vi "zipToxml.vi"(4 "passYield":dbl, 5 "DBSet":T1, 6 "uploadPath":path, 7 "successxmlpath":path, 8 "转换失败路径":path, 9 "目标路径":path, 10 "status msg ref":refnum<vi>, 11 "path":path caption="zip path") -> ()   [LabVIEW 2011]
panel:
  out "customerPN":string
  out "usedSN":string
  out "result":string
  out "upload":bool
  out "archive name out":path
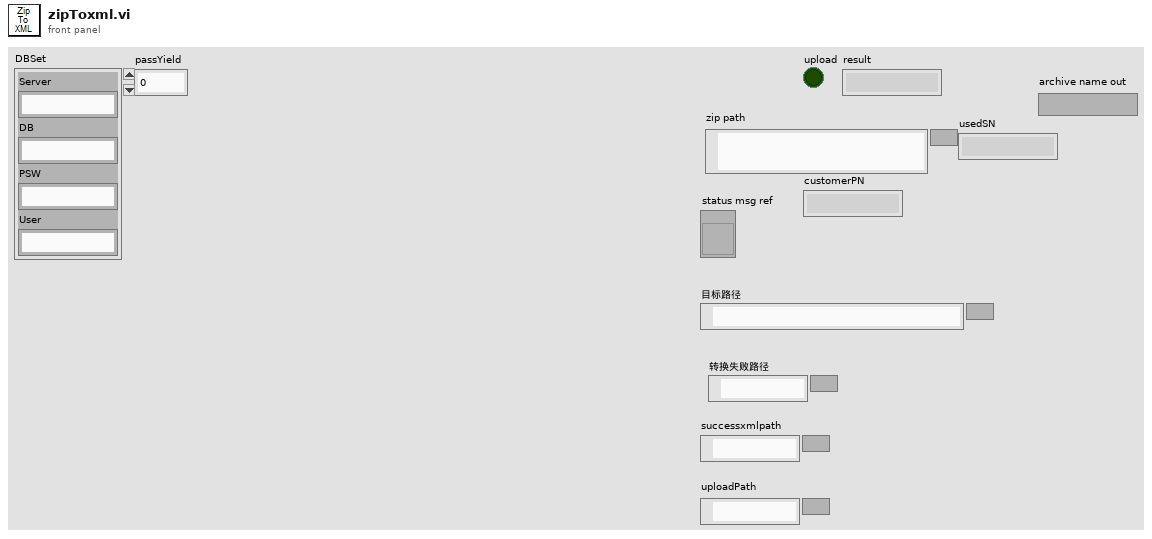
[diagram p1: front panel]
types:
  T1 = cluster{"Server":string, "DB":string, "PSW":string, "User":string}
  T2 = typedef "TDD.ctl" = cluster{"show_Cable Point":dbl[], "show_Terminal Point":dbl[], "show_impspec":string[]}
  T3 = typedef "xml_detail.ctl" = cluster{"FileVersion":string, "FileName":string, "customerPN":string, "usedSN":string, "test time":string[], "testResult":bool}
  T4 = typedef "sSpec.ctl" = cluster{"itemName":string, "upperLimit":dbl[], "lowerLimit":dbl[], "testResult":string, "result":bool}
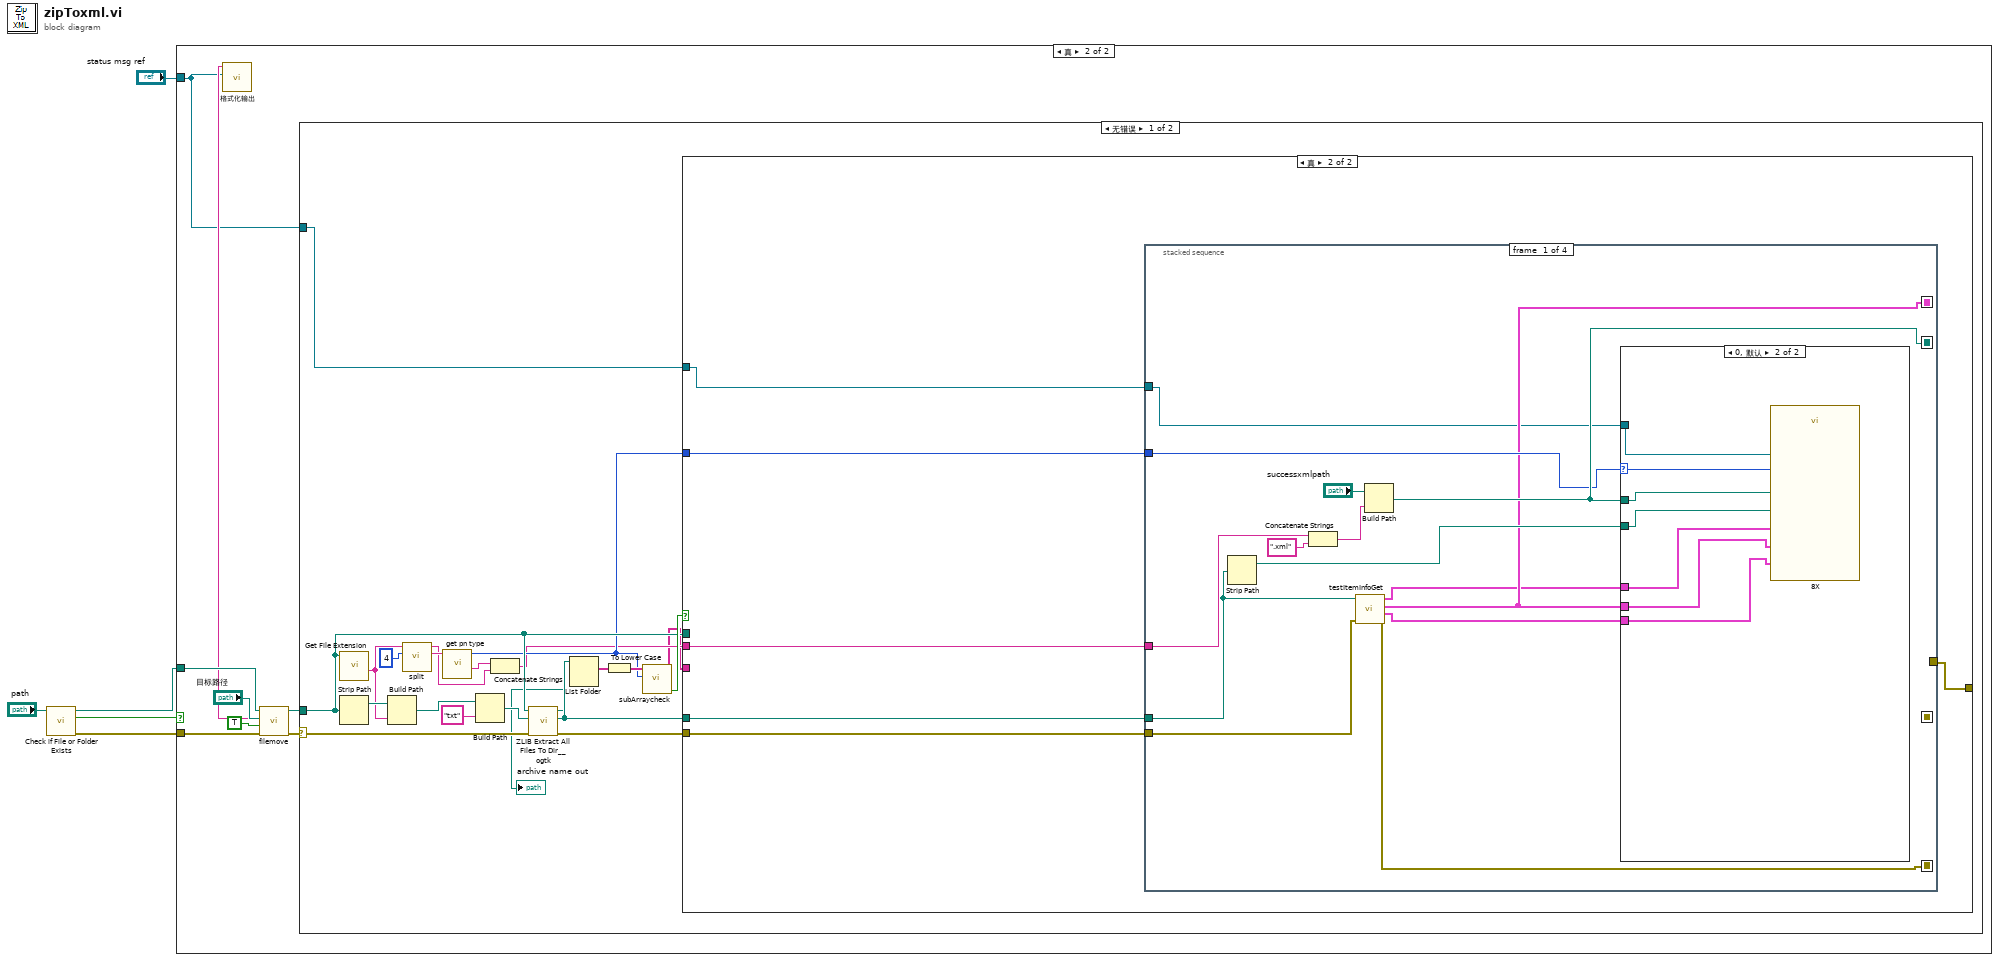
[diagram p0: block diagram]
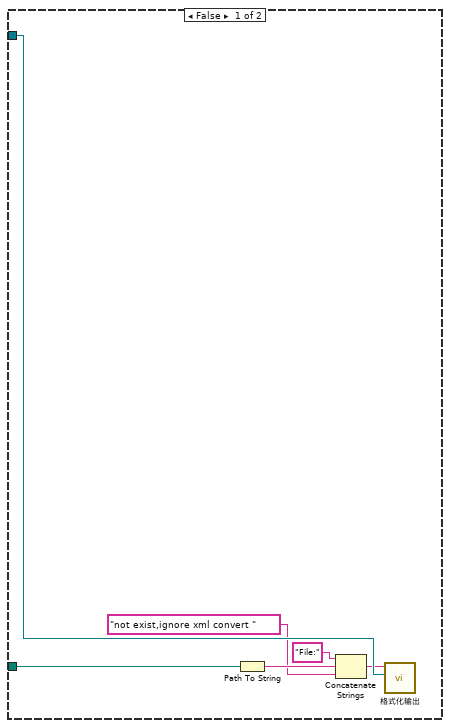
[diagram p2: hidden frame]
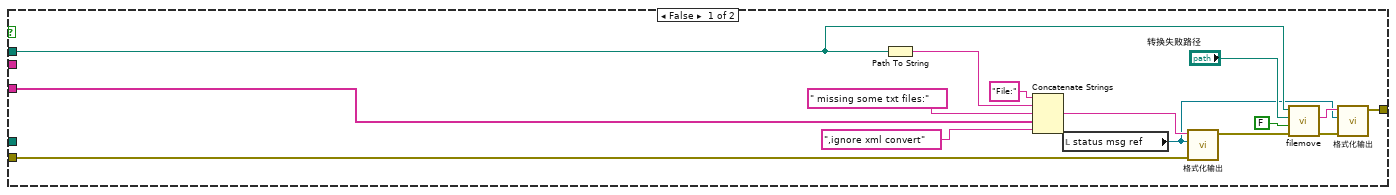
[diagram p3: hidden frame]
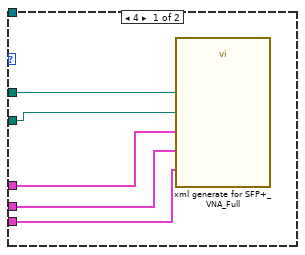
[diagram p4: hidden frame]
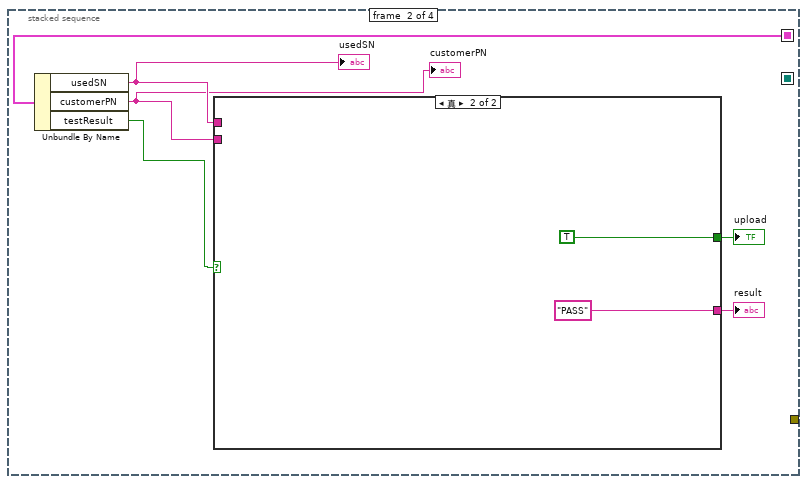
[diagram p5: hidden frame]
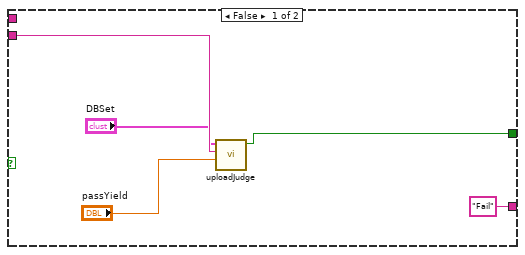
[diagram p6: hidden frame]
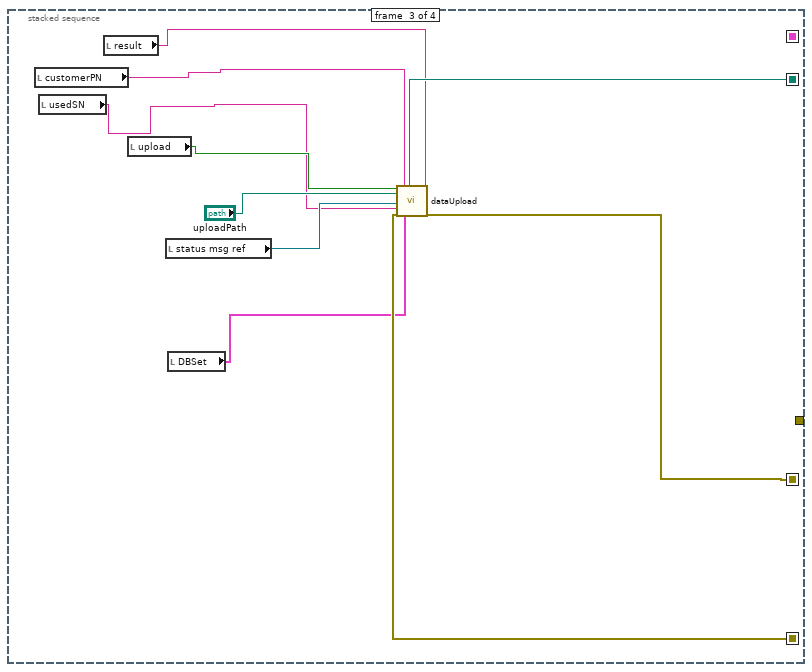
[diagram p7: hidden frame]
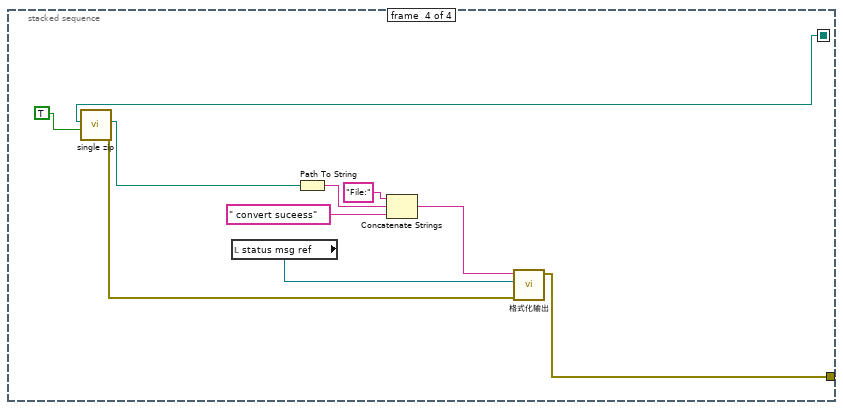
[diagram p8: hidden frame]
diagram:
  n1 = call <vilib>:"Check if File or Folder Exists.vi"("path"="path") -> ("error out"=w2:errorcluster, "file or folder exists?"=w5:bool, "dup path"=w4:path)  [unwired: 8 in]
  n2 = case shown="真" w5 {
    tunnel: w4 -> [w10 w19]
    tunnel: "status msg ref" -> [w11 w12]
    tunnel: w2 -> [_ w13]
    frame False {
      n3 = Path To String(path=w10) -> (string=w8:string)
      n4 = Concatenate Strings("File:" ("字符串"), w8, "not exist,ignore xml convert " ("字符串")) -> (w6:string)
      n5 = call "格式化输出.vi"("字符串引用"=w11, "字符串"=w6) -> ()  [unwired: 9 in, 1 out]
    }
    frame True {
      n6 = call "filemove.vi"("错误输入"=w13, "清空"=TRUE, "目标路径"="目标路径", "源路径"=w19) -> ("错误输出"=w18:errorcluster, "msg"=w15:string, "新路径"=w17:path)  [unwired: 5 in]
      n7 = call "格式化输出.vi"("字符串引用"=w12, "字符串"=w15) -> ()  [unwired: 9 in, 1 out]
      n8 = case shown="无错误" w18 {
        selector: w18 -> [w32 _]
        tunnel: w17 -> [w33 _]
        tunnel: w12 -> [w20 _]
        frame No Error {
          n9 = call <nishared>:"Get File Extension.vi"("file"=w33) -> ("filename without extension"=w29:string)  [unwired: 7 in, 3 out]
          n10 = Strip Path(path=w33) -> (stripped path=w40:path)  [unwired: 1 out]
          n11 = Build Path(base path=w40, name or relative path=w29) -> (appended path=w39:path)
          n12 = call "split.vi"("长度"=4, "source"=w29) -> ("left"=w27:string, "right"=w22:string)  [unwired: 8 in]
          n13 = call "get pn type.vi"("字符串"=w27) -> ("type adder"=w23:string, "type"=w26:i32)  [unwired: 9 in]
          n14 = Build Path(base path=w39, name or relative path="txt" ("名称或相对路径")) -> (appended path=w37:path)
          n15 = Concatenate Strings(w23, w22) -> (w24:string)
          n16 = call <userlib>:"ZLIB Extract All Files To Dir__ogtk.vi"("error in (no error)"=w32, "root directory (archive name without ending)"=w37, "archive name (file dialog)"=w33) -> ("error out"=w31:errorcluster, "root directory out"=w36:path, "archive name out"=→"archive name out":path)  [unwired: 6 in]
          n17 = List Folder(path=w36) -> (filenames=w30:string[])  [unwired: 3 in, 3 out]
          n18 = To Lower Case(string=w30) -> (all lower case string=w35:string[])
          n19 = call "subArraycheck.vi"("type"=w26, "source"=w35) -> ("is in?"=w34:bool, "diff element"=w21:string[])  [unwired: 8 in]
          n20 = case shown="真" w34 {
            tunnel: w24 -> [_ w61]
            tunnel: w36 -> [_ w60]
            tunnel: w33 -> [w53 _]
            tunnel: w31 -> [w44 w59]
            tunnel: [w43 w57] -> _
            tunnel: w26 -> [_ w58]
            tunnel: w21 -> [w42 _]
            tunnel: w20 -> [_ w56]
            frame False {
              n21 = Path To String(path=w53) -> (string=w51:string)
              n22 = Concatenate Strings("File:" ("字符串"), w51, " missing some txt files:" ("字符串"), w42, ",ignore xml convert") -> (w49:string)
              n23 = local read "status msg ref"() -> (w47:refnum<vi>)
              n24 = call "格式化输出.vi"("错误输入（无错误）"=w44, "字符串引用"=w47, "字符串"=w49) -> ("错误输出"=w46:errorcluster)  [unwired: 8 in]
              n25 = call "filemove.vi"("错误输入"=w46, "清空"=FALSE, "目标路径"="转换失败路径", "源路径"=w53) -> ("错误输出"=w45:errorcluster, "msg"=w48:string)  [unwired: 5 in, 1 out]
              n26 = call "格式化输出.vi"("错误输入（无错误）"=w45, "字符串引用"=w47, "字符串"=w48) -> ("错误输出"=w43:errorcluster)  [unwired: 8 in]
            }
            frame True {
              n27 = stacked-sequence {
                seq-local: [w71 _ _ _] -> [_ _ w106 w120]
                seq-local: [w63 _ _ _] -> [_ _ w109 _]
                seq-local: [_ _ w108 _] -> [_ _ _ _]
                seq-local: [w67 _ _ _] -> [_ w89 _ _]
                tunnel: w61 -> [w74 _ _ _]
                tunnel: w60 -> [w68 _ _ _]
                tunnel: w59 -> [w64 _ _ _]
                tunnel: w58 -> [w69 _ _ _]
                tunnel: [_ _ _ w111] -> w57
                tunnel: w56 -> [w62 _ _ _]
                frame #0 {
                  n28 = Strip Path(path=w68) -> (stripped path=w75:path)  [unwired: 1 out]
                  n29 = Concatenate Strings(w74, ".xml" ("字符串")) -> (w72:string)
                  n30 = call "testItemInfoGet.vi"("error in (no error)"=w64, "basePath"=w68) -> ("error out"=w63:errorcluster, "TDD"=w65:T2, "xml_detail"=w67:T3, "singleItemInfo"=w66:T4[])  [unwired: 6 in]
                  n31 = Build Path(base path="successxmlpath", name or relative path=w72) -> (appended path=w71:path)
                  n32 = case shown="0, 默认" w69 {
                    selector: w69 -> [_ w87]
                    tunnel: w75 -> [w79 w85]
                    tunnel: w71 -> [w80 w86]
                    tunnel: w67 -> [w77 w83]
                    tunnel: w66 -> [w78 w84]
                    tunnel: w65 -> [w76 w82]
                    tunnel: w62 -> [_ w81]
                    frame 4 {
                      n33 = call "xml generate for SFP+_VNA_Full.vi"("xmlPath"=w80, "txtPath"=w79, "singleItemInfo"=w78, "xml_detail"=w77, "TDD"=w76) -> ()  [unwired: 11 in]
                    }
                    frame 0, Default {
                      n34 = call "8X.vi"("xml path"=w86, "type"=w87, "txtPath"=w85, "singleItemInfo"=w84, "xml_detail"=w83, "TDD"=w82, "StatusRef"=w81) -> ()  [unwired: 9 in]
                    }
                  }
                }
                frame #1 {
                  n35 = Unbundle By Name(w89) -> ("usedSN"=w93:string, "customerPN"=w92:string, "testResult"=w88:bool)
                  "usedSN" <- w93
                  "customerPN" <- w92
                  n36 = case shown="真" w88 {
                    tunnel: [w97 TRUE] -> w91
                    tunnel: ["Fail" "PASS"] -> w90
                    tunnel: w93 -> [_ _]
                    tunnel: w92 -> [w95 _]
                    frame False {
                      n37 = call "uploadJudge.vi"("passYield"="passYield", "pn"=w95, "DBSet"="DBSet") -> ("upload"=w97:bool)  [unwired: 8 in]
                    }
                    frame True {
                    }
                  }
                  "upload" <- w91
                  "result" <- w90
                }
                frame #2 {
                  n38 = local read "customerPN"() -> (w103:string)
                  n39 = local read "usedSN"() -> (w102:string)
                  n40 = local read "result"() -> (w104:string)
                  n41 = local read "upload"() -> (w105:bool)
                  n42 = local read "status msg ref"() -> (w107:refnum<vi>)
                  n43 = local read "DBSet"() -> (w101:T1)
                  n44 = call "dataUpload.vi"("upload"=w105, "uploadpath"="uploadPath", "status msg ref"=w107, "sn"=w102, "错误输入（无错误）"=w109, "pn"=w103, "DBSet"=w101, "xmlPath"=w106, "result"=w104) -> ("错误输出"=w108:errorcluster)  [unwired: 10 in]
                }
                frame #3 {
                  n45 = call "single zip.vi"("del source?"=TRUE, "source file path"=w120) -> ("error out"=w112:errorcluster, "output zip"=w114:path)  [unwired: 8 in]
                  n46 = local read "status msg ref"() -> (w113:refnum<vi>)
                  n47 = Path To String(path=w114) -> (string=w117:string)
                  n48 = Concatenate Strings("File:" ("字符串"), w117, " convert suceess" ("字符串")) -> (w115:string)
                  n49 = call "格式化输出.vi"("错误输入（无错误）"=w112, "字符串引用"=w113, "字符串"=w115) -> ("错误输出"=w111:errorcluster)  [unwired: 8 in]
                }
              }
            }
          }
        }
        frame Error {
        }
      }
    }
  }
